vi "Pipeline 2ch.vi"(10 "data in":T1[](array[typedef]), 11 "data in":T1[](array[typedef])) -> (2 "data out":T1[](array[typedef]), 3 "data out":T1[](array[typedef]))   [LabVIEW 2025, in "niUSRP Rx DSP v2 FPGA.lvclass"]
uses:
  niUSRP Rx DSP v2 FPGA.lvclass
  niUSRP Rx DSP v2 FPGA.lvclass/niUSRP Rx DSP v2 FPGA.ctl
  <instrlib>/_niInstr/DSP/v1/Shared/Public/IQ Data.ctl
  <instrlib>/_niInstr/DSP/v1/Shared/niInstr DSP v1 Shared.lvlib
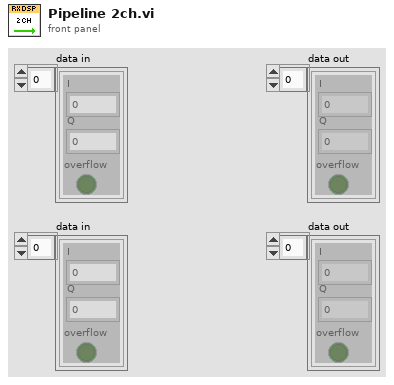
[diagram p1: front panel]
types:
  T1 = typedef "niInstr DSP v1 Shared.lvlib/IQ Data.ctl" = cluster{"I":fxp<+/-,18,1>, "Q":fxp<+/-,18,1>, "overflow":bool}
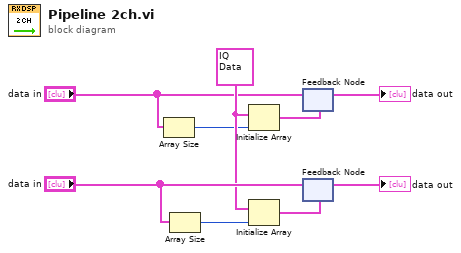
[diagram p0: block diagram]
diagram:
  w6 = T1 {"I"=0.0, "Q"=0.0, "overflow"=FALSE} ("data")
  n1 = Array Size(array="data in") -> (size(s)=w4:i32)
  n2 = Array Size(array="data in") -> (size(s)=w5:i32)
  n3 = Initialize Array(w6, w4) -> (w9:T1[])
  n4 = Initialize Array(w6, w5) -> (w8:T1[])
  n5 = feedback #1(w9) -> (→"data out":T1[])
  n6 = feedback-in #1("data in") -> ()
  n7 = feedback #2(w8) -> (→"data out":T1[])
  n8 = feedback-in #2("data in") -> ()
